vi "Stop or Exit in Message Queue.vi"(8 "error in (no error)":errorcluster, 11 "queue":refnum<queue>) -> (0 "error out":errorcluster, 3 "x .or. y?":bool)   [LabVIEW 2017, in "Message Queue.lvlib"]
uses:
  Message Queue.lvlib
  Message Cluster.ctl
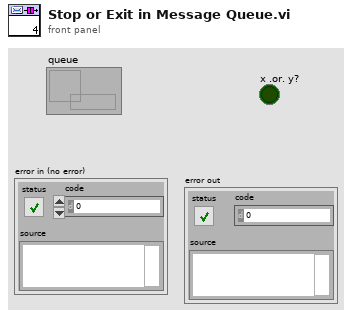
[diagram p1: front panel]
types:
  T1 = typedef "Message Queue.lvlib/Message Cluster.ctl" = cluster{"Message":string, "Message Data":variant}
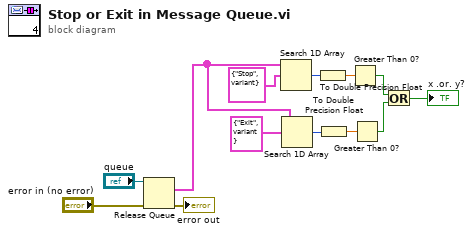
[diagram p0: block diagram]
diagram:
  n1 = Release Queue(queue="queue", error in (no error)="error in (no error)") -> (remaining elements=w12:T1[], error out=→"error out":errorcluster)  [unwired: 1 in, 1 out]
  n2 = Search 1D Array(1D array=w12, element=T1 {"Message"="Stop", "Message Data"=variant} ("remaining elements")) -> (index of element=w10:i32)  [unwired: 1 in]
  n3 = Search 1D Array(1D array=w12, element=T1 {"Message"="Exit", "Message Data"=variant} ("remaining elements")) -> (index of element=w9:i32)  [unwired: 1 in]
  n4 = To Double Precision Float(number=w10) -> (double precision float=w8:dbl)
  n5 = To Double Precision Float(number=w9) -> (double precision float=w7:dbl)
  n6 = Greater Than 0?(x=w8) -> (x > 0?=w6:bool)
  n7 = Greater Than 0?(x=w7) -> (x > 0?=w5:bool)
  n8 = Or(x=w6, y=w5) -> (x .or. y?=→"x .or. y?":bool)
